vi "FTW-TransferClient-Download.vi"(0 "Transfer Client":refnum<class "FTW-TransferClient-S3.lvclass">, 11 "error in":errorcluster) -> (4 "Transfer Client out":refnum<class "FTW-TransferClient-S3.lvclass">, 6 "Data":string, 8 "Download Time":u32 format="%06dmsec", 15 "error out":errorcluster)   [LabVIEW 2014, in "FTW-TransferClient-S3.lvclass"]
uses:
  FTW-TransferClient-S3.lvclass
  FTW-TransferClient.lvclass
panel:
  # "Inputs"
  # "Outputs"
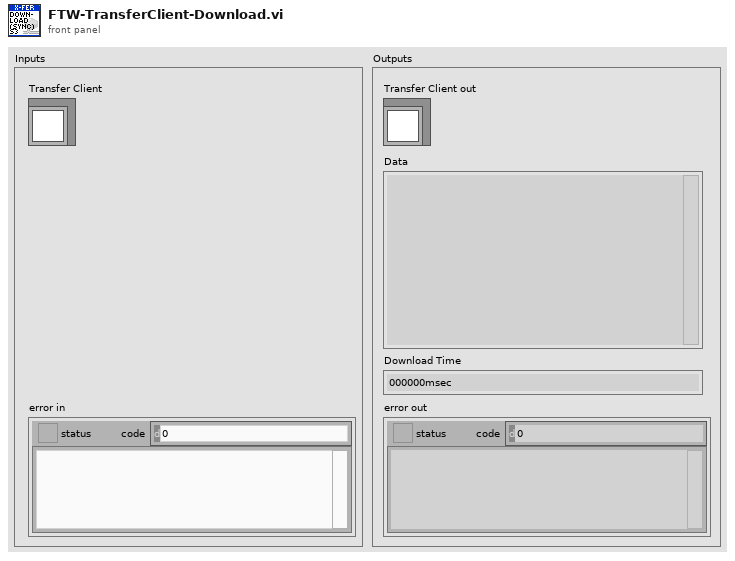
[diagram p1: front panel]
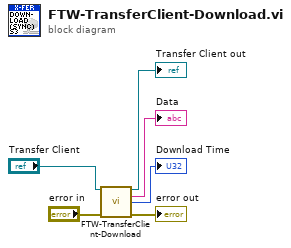
[diagram p0: block diagram]
diagram:
  n1 = call-parent "FTW-TransferClient-Download.vi"("Transfer Client"="Transfer Client", "error in"="error in") -> ("Transfer Client out"=→"Transfer Client out":refnum<class "FTW-TransferClient-S3.lvclass">, "Data"=→"Data":string, "Download Time"=→"Download Time":u32, "error out"=→"error out":errorcluster)  [unwired: 10 in]
